vi "Read Name.vi"(8 "error in (no error)":errorcluster, 11 "Command in":refnum<class "Command.lvclass">) -> (0 "error out":errorcluster, 2 "Name":string, 3 "Command out":refnum<class "Command.lvclass">)   [LabVIEW 2013, in "Command Processor.lvlib" / "Command.lvlib" / "Command.lvclass"]
uses:
  Command.lvclass
  Command.lvclass/Command.ctl
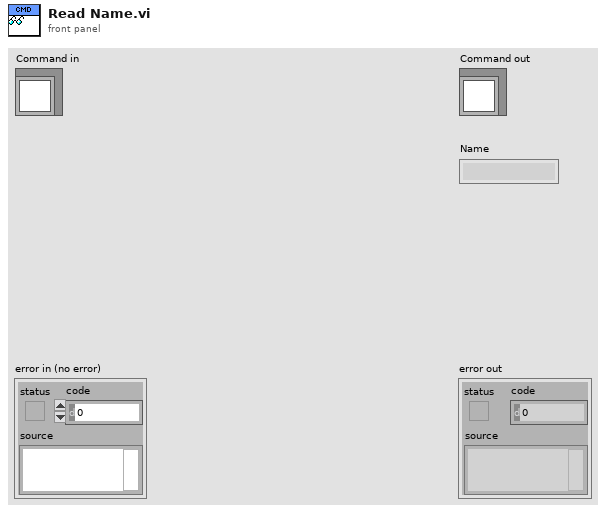
[diagram p1: front panel]
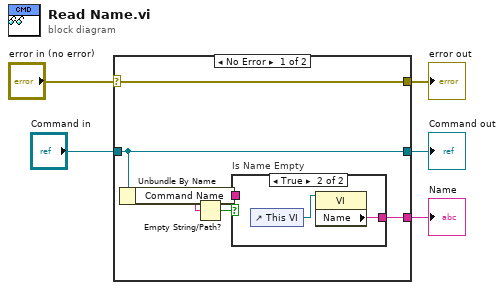
[diagram p0: block diagram]
diagram:
  n1 = case shown="No Error" "error in (no error)" {
    selector: "error in (no error)" -> [w10 w14]
    tunnel: [w10 w14] -> w4
    tunnel: [w9 w15] -> w2
    tunnel: "Command in" -> [w9 w15]
    tunnel: [w6 _] -> w1
    frame No Error {
      n2 = Unbundle By Name(w9) -> ("Command Name"=w7:string)
      n3 = Empty String/Path?(string/path=w7) -> (empty?=w8:bool)
      n4 = case "Is Name Empty" shown="True" w8 {
        tunnel: w7 -> [w11 _]
        tunnel: [w11 w12] -> w6
        frame False {
        }
        frame True {
          n5 = control-ref of="This VI"() -> (w13:refnum<vi>)
          n6 = property class="VI"(reference=w13) -> ("Name"=w12:string)  [unwired: 1 in, 2 out]
        }
      }
    }
    frame Error {
    }
  }
  "error out" <- w4
  "Command out" <- w2
  "Name" <- w1
